vi "Configure Input Relative Attenuation.vi"(0 "VISA resource name":refnum<visa-resource-name>, 5 "Platform Slot Number (10)":i16=10 min=-1 max=255, 7 "Relative Attenuation (0:MINimum)":i32(ring) items=["MINimum", "MAXimum", "DEFault", "User Defined Value"], 9 "User Defined Relative Attenuation Value (-4.4497)":dbl=-4.44967 format="%_5g", 11 "error in (no error)":errorcluster) -> (4 "VISA resource name out":refnum<visa-resource-name>, 15 "error out":errorcluster)   [LabVIEW 2018, in "LTB-1.lvlib" / "3150.lvlib"]
doc: "Configures the relative attenuation to a specific value, in dB. The valid range of values depends on the type of instrument, the configuration, and the current wavelength. This value is used only when the ATTenuation control mode is active."
uses:
  3150.lvlib
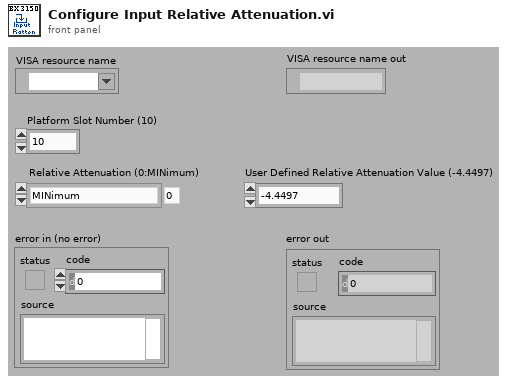
[diagram p1: front panel]
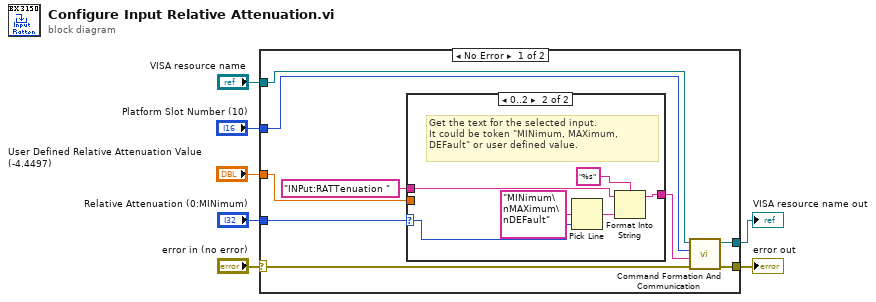
[diagram p0: block diagram]
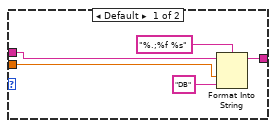
[diagram p2: hidden frame]
diagram:
  n1 = case shown="No Error" "error in (no error)" {
    selector: "error in (no error)" -> [w13 w29]
    tunnel: "VISA resource name" -> [w14 w28]
    tunnel: [w10 w29] -> w5
    tunnel: "Relative Attenuation (0:MINimum)" -> [w9 _]
    tunnel: "Platform Slot Number (10)" -> [w12 _]
    tunnel: [w11 w28] -> w2
    tunnel: "User Defined Relative Attenuation Value (-4.4497)" -> [w8 _]
    frame No Error {
      n2 = case shown="0..2" w9 {
        selector: w9 -> [_ w24]
        tunnel: "INPut:RATTenuation " ("Command") -> [w20 w23]
        tunnel: [w19 w22] -> w15
        tunnel: w8 -> [w17 _]
        frame Default {
          n3 = Format Into String(format string="%.;%f %s", initial string=w20, w17, "DB") -> (resulting string=w19:string)  [unwired: 1 in, 1 out]
        }
        frame 0..2 {
          # "Get the text for the selected input.\nIt could be token \"MINimum, MAXimum,\nDEFault\" or user defined value."
          n4 = Pick Line(multi-line string="MINimum\nMAXimum\nDEFault", line index=w24) -> (output string=w25:string)  [unwired: 1 out]
          n5 = Format Into String(format string="%s", initial string=w23, w25) -> (resulting string=w22:string)  [unwired: 1 in, 1 out]
        }
      }
      n6 = call "Command Formation And Communication.vi"("error in (no error)"=w13, "Command"=w15, "Platform Slot Number"=w12, "VISA resource name"=w14) -> ("error out"=w10:errorcluster, "VISA resource name out"=w11:refnum<visa-resource-name>)  [unwired: 6 out]
    }
    frame Error {
    }
  }
  "VISA resource name out" <- w2
  "error out" <- w5
